vi "CoerceForTDT Read.vi"(4 "error in (no error)":errorcluster, 6 "Container State":T5, 7 "Display State In":T1) -> (0 "error out":errorcluster, 2 "Value":bool, 3 "Display State Out":T1)   [LabVIEW 2020, in "SignalManager.xctl"]
uses:
  SignalManager.xctl
  <vilib>/_xctls/Container State.ctl
  State.ctl
  Utility VIs/Controls/KListboxEx/Events.ctl
  Utility VIs/Controls/KListboxEx/Event Action.ctl
  PeriodDisplay.ctl
  Events.ctl
  Event Data.ctl
  <vilib>/_xctls/XControlSupport.lvlib
  Utility VIs/Controls/KListboxEx/KListboxEx.xctl
panel:
  # "Replace the Value Indicator below with an Indicator of desired type.\nDo not remove this Indicator or the others from the connector pane. \nDo not change the connector pane pattern.\nThe Value Indicator should always be the second terminal from top on the output side in the connector pane."
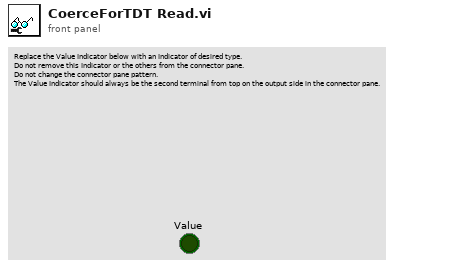
[diagram p1: front panel]
types:
  T1 = typedef "SignalManager.xctl/State.ctl" = cluster{"Channels":T2, "Destinations":string[], "action":string, "EventReg":refnum<event-registration>, "selectedChan":i32, "Period Display":T3, "Events":T4, "Fs (Hz)":dbl, "TDT":bool}
  T2 = typedef "KListboxEx.xctl/Events.ctl" = cluster{"Items Changed":refnum<user-event>, "List Changed":refnum<user-event>}
  T3 = typedef "SignalManager.xctl/PeriodDisplay.ctl" = enum16{"Interval", "RepRate", "Both"}
  T4 = typedef "SignalManager.xctl/Events.ctl" = cluster{"Rename":refnum<user-event>}
  T5 = typedef "XControlSupport.lvlib/Container State.ctl" = cluster{"Indicator?":bool, "Run Mode?":bool, " Refnum":refnum<vi>}
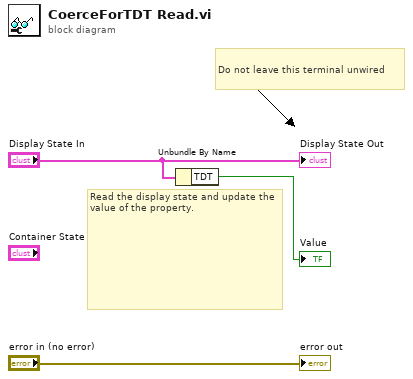
[diagram p0: block diagram]
diagram:
  # "Do not leave this terminal unwired"
  # "Read the display state and update the value of the property."
  n1 = Unbundle By Name("Display State In") -> ("TDT"=→"Value":bool)
  "error out" <- "error in (no error)"
  "Display State Out" <- "Display State In"
